vi "RFH-View-sort_by_name_comp.vi"() -> ()   [LabVIEW 2020, in "RFH-Reflection_File_Handler.lvlib"]
uses:
  RFH-Reflection_File_Handler.lvlib
  RFH-common_data_format.ctl
  c8c21ec7-ed02-4f39-bd47-49b2af03b8e9.vi
  <vilib>/Comparison/Less/Less Functor/Less Functor.lvclass
panel:
  out "sorted array":string[](array[string])
  out "Array":string[](array[string])
  out "Reflection Imag 2":T1(graph)
  in  "stop":bool
  out "Reflection Imag":T1(graph)
  in  "Folder Path":path=path "C:/projects/Universitet/Master/data/Real Test - First libreVNA test with calibration file/Converted Data"
  out "Reflection Real":T1(graph)
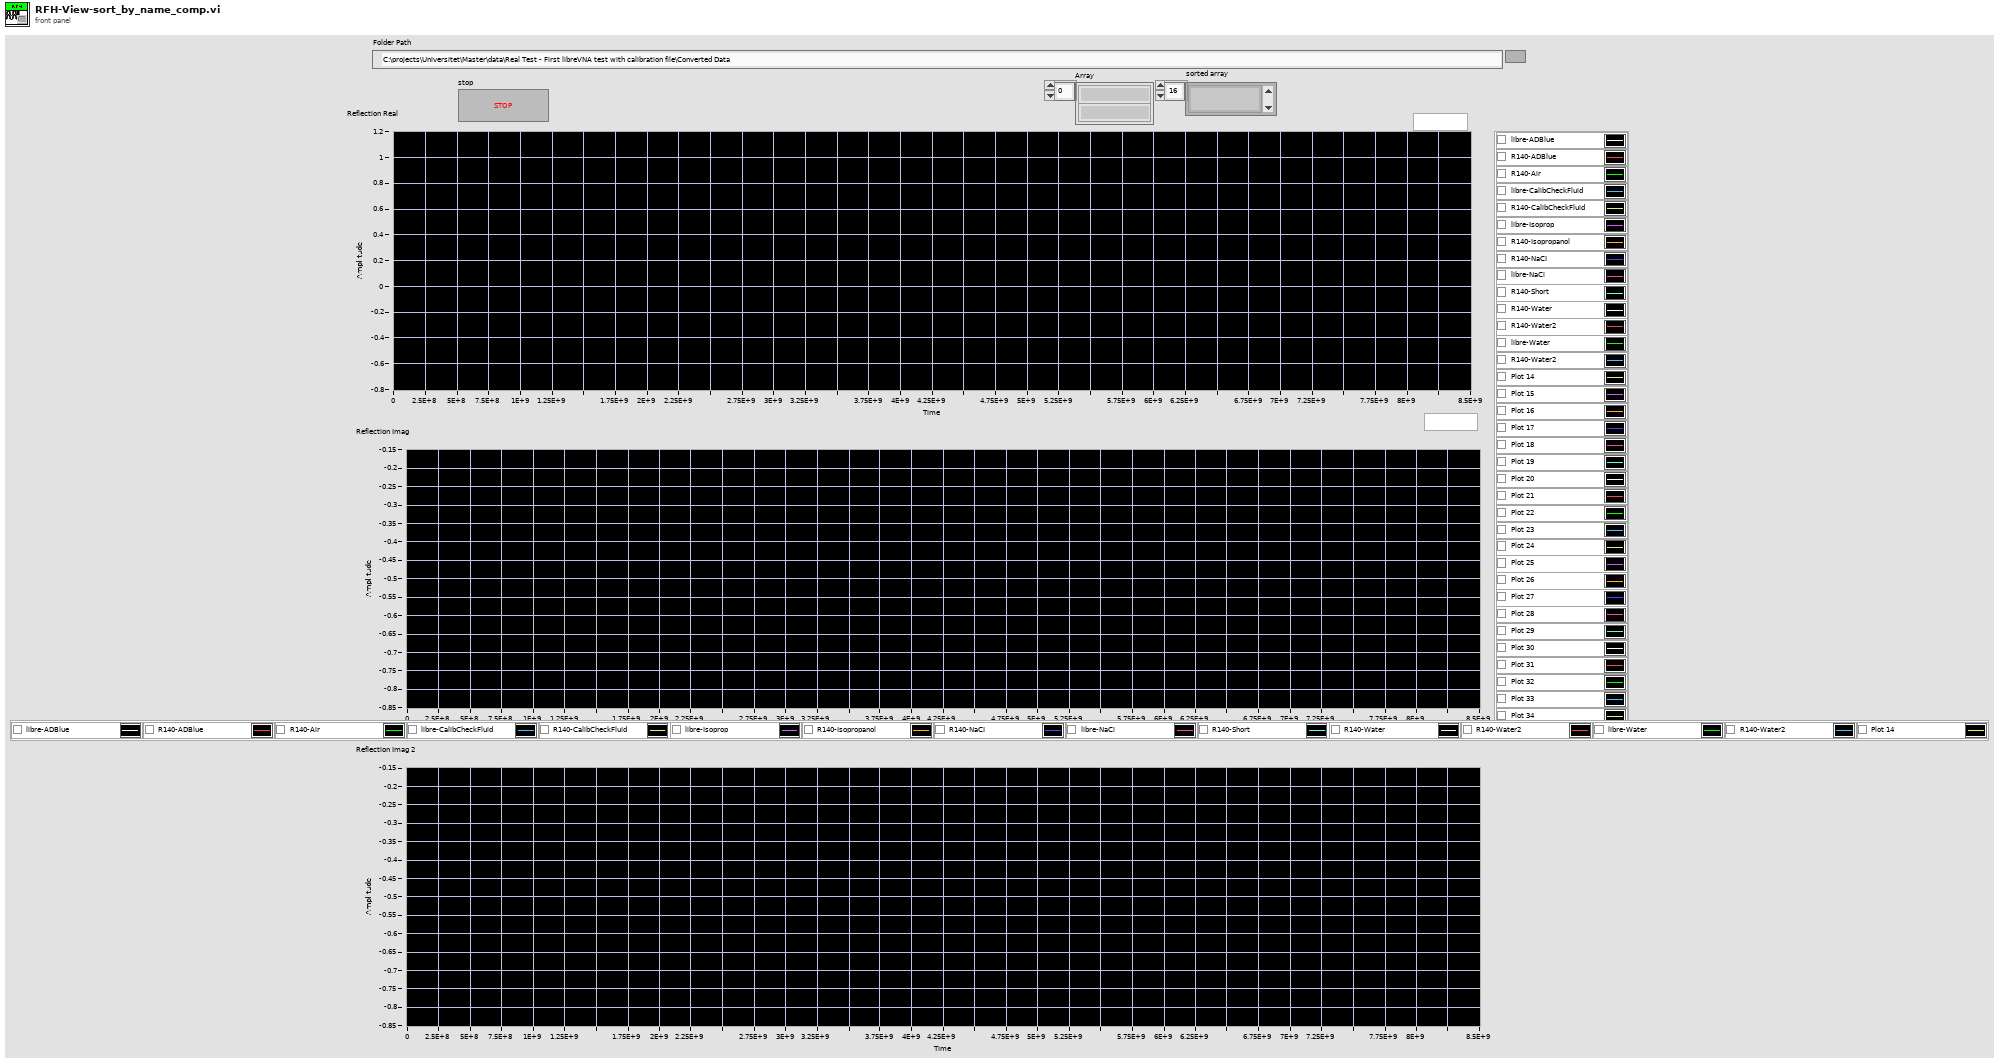
[diagram p1: front panel]
types:
  T1 = cluster{"Frequency":dbl[], "Reflection'":dbl[]}[]
  T2 = cluster{"Reflection Real":cluster{"Frequency":dbl[], "Reflection'":dbl[]}[], "Reflection Imag":cluster{"Frequency":dbl[], "Reflection'":dbl[]}[], "ref2":cluster{"Frequency":dbl[], "Reflection''":dbl[]}[]}
  T3 = typedef "RFH-Reflection_File_Handler.lvlib/RFH-common_data_format.ctl" = cluster{"Frequency":dbl[], "Reflection'":dbl[], "Reflection''":dbl[], "Permativity'":dbl[], "Permativity''":dbl[]}
  T4 = cluster{"XY graph":refnum<vi>[], "data map":map{string, cluster{"filename without extension":string, "Common Format":T3}}, "sorted order":string[]}
  T5 = cluster{"filename without extension":string, "Common Format":T3}
  T6 = map{string, cluster{"filename without extension":string, "Common Format":T3}}
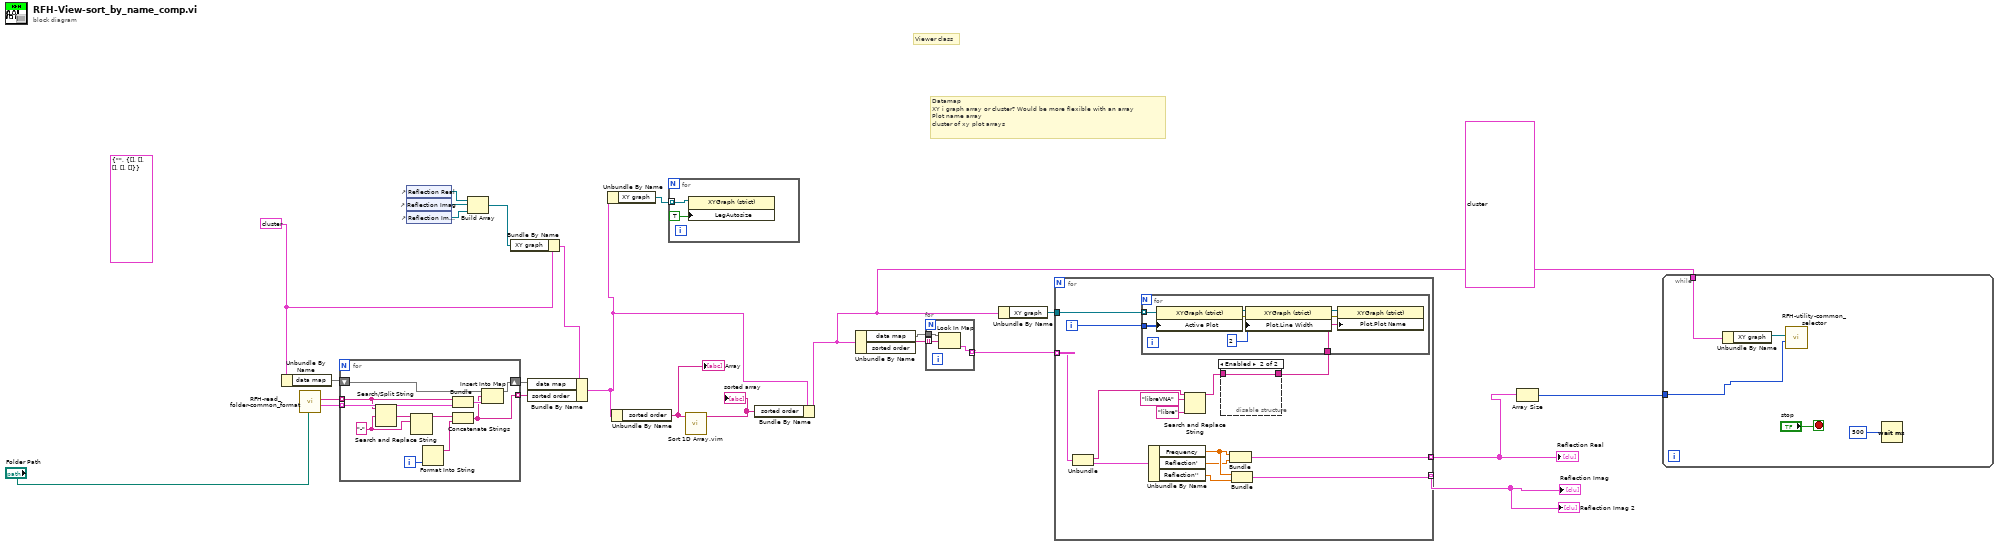
[diagram p0: block diagram]
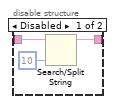
[diagram p2: hidden frame]
diagram:
  (unwired) T2 data[363132B]
  w14 = T4 {"XY graph"=[], "data map"={}, "sorted order"=[]}
  (unwired) T5 {"filename without extension"="", "Common Format"={"Frequency"=[], "Reflection'"=[], "Reflection''"=[], "Permativity'"=[], "Permativity''"=[]}} ("output cluster")
  # "Datamap\nXY i graph array or cluster? Would be more flexible with an array\nPlot name array\ncluster of xy plot arrays"
  # "Viewer class"
  n1 = Unbundle By Name(w14) -> ("data map"=w11:T6)
  n2 = call "RFH-read_folder-common_format.vi"("Folder Path"="Folder Path") -> ("Data"=w16:T3[], "Names"=w17:string[])  [unwired: 8 in, 1 out]
  n3 = for {
    tunnel: w17 -> [w26] mode=indexing
    tunnel: [w25] -> w7 mode=indexing
    tunnel: w16 -> [w33] mode=indexing
    shift-right: [w30] -> w9
    shift-left: w11 -> [w32]
    i -> [w29]
    w34 = "-" ("search string/char (-)")
    n4 = Search/Split String(string=w26, search string/char (-)=w34) -> (match + rest of string=w35:string)  [unwired: 1 in, 2 out]
    n5 = Search and Replace String(input string=w35, search string=w34) -> (result string=w28:string)  [unwired: 6 in, 3 out]
    n6 = Format Into String(w29) -> (resulting string=w27:string)  [unwired: 3 in, 1 out]
    n7 = Bundle("filename without extension"=w26, "Common Format"=w33) -> (w31:T5)  [unwired: 1 in]
    n8 = Concatenate Strings(w28, w27) -> (w25:string)
    n9 = Insert Into Map(map in=w32, key=w25, value=w31) -> (map out=w30:T6)  [unwired: 2 out]
  }
  n10 = control-ref of="Reflection Real"() -> (w21:refnum<vi>)
  n11 = control-ref of="Reflection Imag"() -> (w20:refnum<vi>)
  n12 = control-ref of="Reflection Imag 2"() -> (w22:refnum<vi>)
  n13 = Build Array(w21, w20, w22) -> (w12:refnum<vi>[])
  n14 = Bundle By Name(cluster=w14, "XY graph"=w12) -> (w10:T4)
  n15 = Bundle By Name(cluster=w10, "data map"=w9, "sorted order"=w7) -> (w2:T4)
  n16 = Unbundle By Name(w2) -> ("XY graph"=w8:refnum<vi>[])
  n17 = Unbundle By Name(w2) -> ("sorted order"=w6:string[])
  "Array" <- w6
  n18 = for {
    tunnel: w8 -> [w36] mode=indexing
    n19 = property on="Property Node" class="XYGraph (strict)"(reference=w36, "LegAutosize"=TRUE ("Legend:Autosize")) -> ()  [unwired: 1 in, 2 out]
  }
  n20 = call "Sort 1D Array.vim"("unsorted array"=w6) -> ("sorted array"=w5:string[])  [unwired: 10 in]
  "sorted array" <- w5
  n21 = Bundle By Name(cluster=w2, "sorted order"=w5) -> (w1:T4)
  n22 = Unbundle By Name(w1) -> ("data map"=w4:T6, "sorted order"=w3:string[])
  n23 = for {
    tunnel: w3 -> [w40] mode=indexing
    tunnel: w4 -> [w39]
    tunnel: [w38] -> w15 mode=indexing
    n24 = Look In Map(map=w39, key=w40) -> (value=w38:T5)  [unwired: 1 in, 1 out]
  }
  n25 = Unbundle By Name(w1) -> ("XY graph"=w13:refnum<vi>[])
  n26 = for {
    tunnel: [w51] -> w19 mode=indexing
    tunnel: [w50] -> w23 mode=indexing
    tunnel: w13 -> [w44]
    tunnel: w15 -> [w43] mode=indexing
    i -> [w49]
    n27 = Unbundle(w43) -> ("filename without extension"=w42:string, "Common Format"=w41:T3)
    n28 = Unbundle By Name(w41) -> ("Frequency"=w54:dbl[], "Reflection'"=w53:dbl[], "Reflection''"=w52:dbl[])
    n29 = Search and Replace String(input string=w42, search string="libreVNA", replace string="libre" ("replace string (\"\")")) -> (result string=w45:string)  [unwired: 5 in, 3 out]
    n30 = disable-structure shown="Enabled" {
      disable-tunnel: [w56 w58] -> w48
      disable-tunnel: w45 -> [w55 w58]
      frame Disabled {
        n31 = Search/Split String(string=w55, offset (0)=10) -> (substring before match=w56:string)  [unwired: 1 in, 2 out]
      }
      frame Enabled {
      }
    }
    n32 = for {
      tunnel: w49 -> [w65]
      tunnel: w48 -> [w62]
      tunnel: w44 -> [w61] mode=indexing
      n33 = property on="Property Node" class="XYGraph (strict)"(reference=w61, "Active Plot"=w65) -> (reference out=w60:refnum<vi>, error out=w66:errorcluster)  [unwired: 1 in]
      n34 = property on="Property Node" class="XYGraph (strict)"(reference=w60, error in=w66, "Plot.Line Width"=u8 2) -> (reference out=w59:refnum<vi>, error out=w64:errorcluster)
      n35 = property on="Property Node" class="XYGraph (strict)"(reference=w59, error in=w64, "Plot.Plot Name"=w62) -> ()  [unwired: 2 out]
    }
    n36 = Bundle("Frequency"=w54, "Reflection'"=w53) -> (w51:cluster{"Frequency":dbl[], "Reflection'":dbl[]})  [unwired: 1 in]
    n37 = Bundle("Frequency"=w54, "Reflection''"=w52) -> (w50:cluster{"Frequency":dbl[], "Reflection''":dbl[]})  [unwired: 1 in]
  }
  "Reflection Real" <- w19
  "Reflection Imag" <- w23
  "Reflection Imag 2" <- w23
  n38 = Array Size(array=w19) -> (size(s)=w18:i32)
  n39 = while {
    tunnel: w18 -> [w70]
    tunnel: w1 -> [w68]
    stop <- "stop" stop-if-true
    n40 = Unbundle By Name(w68) -> ("XY graph"=w67:refnum<vi>[])
    n41 = call "RFH-utility-common_selector.vi"("size(s)"=w70, "XY graph refs"=w67) -> ()  [unwired: 10 in]
    n42 = Wait (ms)(milliseconds to wait=u32 500) -> ()  [unwired: 1 out]
  }
